vi "WriteSelectivePacket.vi"(2 "Filename":string, 3 "NXT":T1={"Hardware"="NXT", "Flattened String"=""}, 4 "Time (MS)":i32, 8 "F:Joysticks T:Buttons":bool, 9 "Encoded Data":string) -> (0 "NXT":T1={"Hardware"="NXT", "Flattened String"=""})   [LabVIEW 2010, in "Packet Recorder.lvlib"]
uses:
  Packet Recorder.lvlib
  <vilib>/NXT/Subs/LVHSConnector.ctl
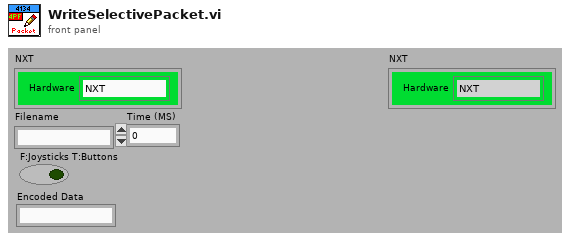
[diagram p1: front panel]
types:
  T1 = typedef "LVHSConnector.ctl" = cluster{"Hardware":string, "Flattened String":string}
  T2 = enum16{"big-endian, network order", "native, host order", "little-endian"}
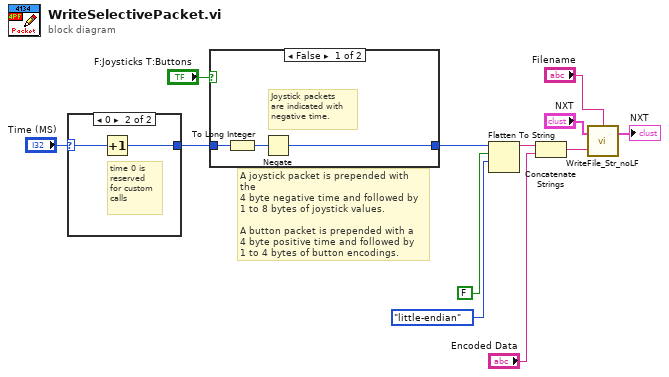
[diagram p0: block diagram]
diagram:
  # "A joystick packet is prepended with the\n4 byte negative time and followed by\n1 to 8 bytes of joystick values.\n\nA button packet is prepended with a\n4 byte positive time and followed by\n1 to 4 bytes of button encodings."
  n1 = case shown="0" "Time (MS)" {
    selector: "Time (MS)" -> [w13 w14]
    tunnel: [w13 w15] -> w1
    frame Default {
    }
    frame 0 {
      # "time 0 is\nreserved\nfor custom\ncalls"
      n2 = Increment(x=w14) -> (x+1=w15:i32)
    }
  }
  n3 = case shown="False" "F:Joysticks T:Buttons" {
    tunnel: w1 -> [w18 w19]
    tunnel: [w16 w19] -> w8
    frame False {
      # "Joystick packets\nare indicated with\nnegative time."
      n4 = To Long Integer(number=w18) -> (32bit integer=w17:i32)
      n5 = Negate(x=w17) -> (-x=w16:i32)
    }
    frame True {
    }
  }
  n6 = Flatten To String(anything=w8, prepend array or string size? (T)=FALSE, byte order (0:big-endian, network order)=T2."little-endian") -> (data string=w5:string)  [unwired: 1 in, 2 out]
  n7 = Concatenate Strings(w5, "Encoded Data") -> (w3:string)
  n8 = call <vilib>:"WriteFile_Str_noLF.vi"("String"=w3, "NXT"="NXT", "Filename"="Filename") -> ("NXT"=→"NXT":T1)  [unwired: 1 in]
